vi "GOOP_ReadDesignPatternIniFile.vi"(8 "error in (no error)":errorcluster, 11 "Path":path) -> (0 "error out":errorcluster, 3 "cluster":T1)   [LabVIEW 2012]
uses:
  <vilib>/Utility/config.llb/Read Key (String).vi
  <vilib>/Utility/config.llb/Read Key (Boolean).vi
  <vilib>/Utility/config.llb/NI_LVConfig.lvlib
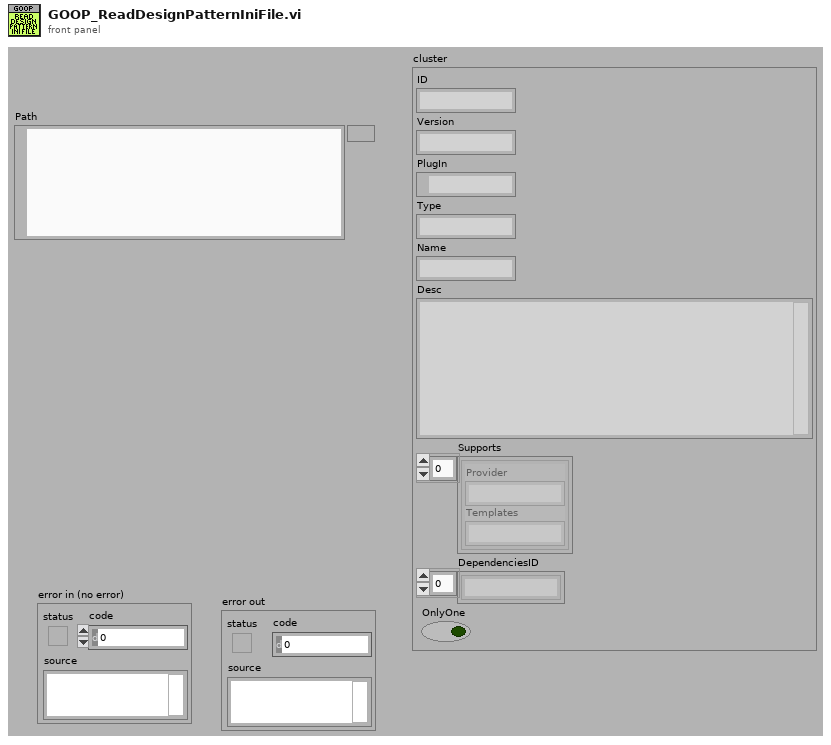
[diagram p1: front panel]
types:
  T1 = cluster{"ID":string, "Version":string, "PlugIn":path, "Type":string, "Name":string, "Desc":string, "Supports":cluster{"Provider":string, "Templates":string}[], "DependenciesID":string[], "OnlyOne":bool}
  T2 = typedef "NI_LVConfig.lvlib/Config Data RefNum.ctl" = refnum<k1>
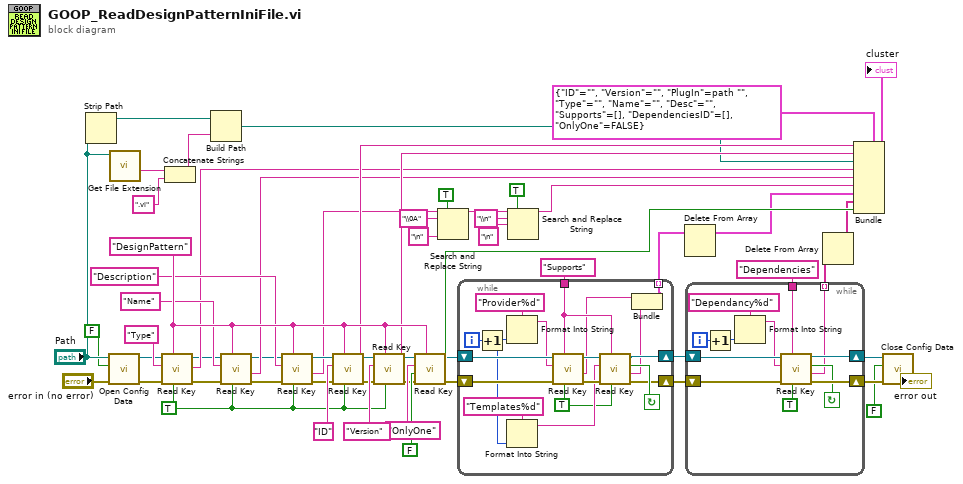
[diagram p0: block diagram]
diagram:
  w35 = TRUE ("read raw string? (F)")
  w50 = "DesignPattern" ("section")
  n1 = Strip Path(path="Path") -> (stripped path=w26:path)  [unwired: 1 out]
  n2 = call <vilib>:"Open Config Data.vi"("error in (no error)"="error in (no error)", "create file if necessary (T)"=FALSE ("create file if necessary? (T)"), "configuration file path"="Path") -> ("error out"=w5:errorcluster, "refnum"=w6:T2)  [unwired: 6 in, 1 out]
  n3 = call <vilib>:"Get File Extension.vi"("file"="Path") -> ("filename without extension"=w27:string)  [unwired: 7 in, 3 out]
  n4 = call-poly <vilib>:"Read Key.vi"("read raw string? (F)"=w35, "section"=w50, "error in (no error)"=w5, "key"="Type", "refnum"=w6) -> ("error out"=w8:errorcluster, "value"=w14:string, "refnum out"=w7:T2)  [unwired: 3 in, 1 out]
  n5 = Concatenate Strings(w27, ".vi" ("string")) -> (w29:string)
  n6 = Build Path(base path=w26, name or relative path=w29) -> (appended path=w30:path)
  n7 = call-poly <vilib>:"Read Key.vi"("read raw string? (F)"=w35, "section"=w50, "error in (no error)"=w8, "key"="Name", "refnum"=w7) -> ("error out"=w10:errorcluster, "value"=w15:string, "refnum out"=w9:T2)  [unwired: 3 in, 1 out]
  n8 = call-poly <vilib>:"Read Key.vi"("read raw string? (F)"=w35, "section"=w50, "error in (no error)"=w10, "key"="Description", "refnum"=w9) -> ("error out"=w32:errorcluster, "value"=w18:string, "refnum out"=w31:T2)  [unwired: 3 in, 1 out]
  n9 = call-poly <vilib>:"Read Key.vi"("read raw string? (F)"=w35, "section"=w50, "error in (no error)"=w32, "key"="ID", "refnum"=w31) -> ("error out"=w34:errorcluster, "value"=w38:string, "refnum out"=w33:T2)  [unwired: 3 in, 1 out]
  n10 = call-poly <vilib>:"Read Key.vi"("read raw string? (F)"=w35, "section"=w50, "error in (no error)"=w34, "key"="Version", "refnum"=w33) -> ("error out"=w46:errorcluster, "value"=w47:string, "refnum out"=w48:T2)  [unwired: 3 in, 1 out]
  n11 = call-poly <vilib>:"Read Key.vi"("section"=w50, "error in (no error)"=w46, "default value"=FALSE ("create file if necessary? (T)"), "key"="OnlyOne", "refnum"=w48) -> ("error out"=w53:errorcluster, "value"=w54:bool, "refnum out"=w52:T2)  [unwired: 3 in, 1 out]
  n12 = Search and Replace String(replace all?=TRUE ("ignore case? (F)"), input string=w18, search string="\\0A", replace string="\n" ("replace string (\"\")")) -> (result string=w57:string)  [unwired: 4 in, 3 out]
  n13 = while {
    shift-right: [w65] -> w39
    shift-left: w53 -> [w76]
    shift-right: [w64] -> w40
    shift-left: w52 -> [w77]
    tunnel: "Supports" ("section") -> [w73]
    tunnel: [w61] -> w22 mode=indexing
    i -> [w71]
    stop <- w66 continue-if-true
    w67 = TRUE ("read raw string? (F)")
    n14 = Increment(x=w71) -> (x+1=w69:i32)
    n15 = Format Into String(format string="Provider%d", w69) -> (resulting string=w70:string)  [unwired: 2 in, 1 out]
    n16 = Format Into String(format string="Templates%d", w69) -> (resulting string=w68:string)  [unwired: 2 in, 1 out]
    n17 = call-poly <vilib>:"Read Key.vi"("read raw string? (F)"=w67, "section"=w73, "error in (no error)"=w76, "key"=w70, "refnum"=w77) -> ("error out"=w75:errorcluster, "value"=w63:string, "refnum out"=w74:T2)  [unwired: 3 in, 1 out]
    n18 = call-poly <vilib>:"Read Key.vi"("read raw string? (F)"=w67, "section"=w73, "error in (no error)"=w75, "key"=w68, "refnum"=w74) -> ("error out"=w65:errorcluster, "value"=w62:string, "found?"=w66:bool, "refnum out"=w64:T2)  [unwired: 3 in]
    n19 = Bundle("value"=w63, "value"=w62) -> (w61:cluster{"value":string, "value":string})  [unwired: 1 in]
  }
  n20 = Search and Replace String(replace all?=TRUE ("ignore case? (F)"), input string=w57, search string="\\n", replace string="\n" ("replace string (\"\")")) -> (result string=w58:string)  [unwired: 4 in, 3 out]
  n21 = Delete From Array(array=w22) -> (array with subset deleted=w23:cluster{"value":string, "value":string}[])  [unwired: 2 in, 1 out]
  n22 = while {
    shift-right: [w82] -> w42
    shift-left: w39 -> [w88]
    shift-right: [w81] -> w41
    shift-left: w40 -> [w89]
    tunnel: [w79] -> w43 mode=indexing
    tunnel: "Dependencies" ("section") -> [w78]
    i -> [w86]
    stop <- w80 continue-if-true
    n23 = Increment(x=w86) -> (x+1=w84:i32)
    n24 = Format Into String(format string="Dependancy%d", w84) -> (resulting string=w85:string)  [unwired: 2 in, 1 out]
    n25 = call-poly <vilib>:"Read Key.vi"("read raw string? (F)"=TRUE, "section"=w78, "error in (no error)"=w88, "key"=w85, "refnum"=w89) -> ("error out"=w82:errorcluster, "value"=w79:string, "found?"=w80:bool, "refnum out"=w81:T2)  [unwired: 3 in]
  }
  n26 = Delete From Array(array=w43) -> (array with subset deleted=w44:string[])  [unwired: 2 in, 1 out]
  n27 = Bundle(cluster=T1 {"ID"="", "Version"="", "PlugIn"=path "", "Type"="", "Name"="", "Desc"="", "Supports"=[], "DependenciesID"=[], "OnlyOne"=FALSE}, "ID"=w38, "Version"=w47, "PlugIn"=w30, "Type"=w14, "Name"=w15, "Desc"=w58, "Supports"=w23, "DependenciesID"=w44, "OnlyOne"=w54) -> (→"cluster":T1)
  n28 = call <vilib>:"Close Config Data.vi"("error in (no error)"=w42, "write file if changed (T)"=FALSE ("write configuration file? (T)"), "refnum"=w41) -> ("error out"=→"error out":errorcluster)  [unwired: 7 in, 1 out]
